vi "Generate API VI.vi"(7 "Highlight changes?":bool=TRUE, 8 "error in (no error)":errorcluster, 9 "class path":path, 10 "API Message":string) -> (0 "error out":errorcluster)   [LabVIEW 2020, in "Method Generation.lvlib" / "API VI Generator.lvclass"]
uses:
  API VI Generator.lvclass
  API VI Generator.lvclass/API VI Generator.ctl
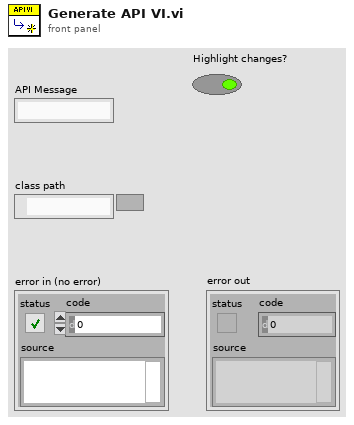
[diagram p1: front panel]
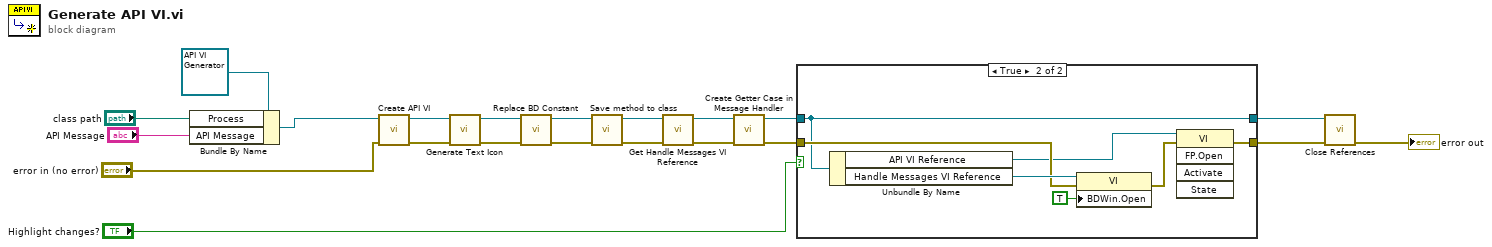
[diagram p0: block diagram]
diagram:
  n1 = Bundle By Name(cluster=refnum<class "API VI Generator.lvclass"> refnum ("New Getter Dialog In"), "Process"="class path", "API Message"="API Message") -> (w17:refnum<class "API VI Generator.lvclass">)
  n2 = call "Create API VI.vi"("error in (no error)"="error in (no error)", "Setter Generator In"=w17) -> ("error out"=w21:errorcluster, "Setter Generator Out"=w2:refnum<class "API VI Generator.lvclass">)  [unwired: 8 in]
  n3 = call "Generate Text Icon.vi"("error in (no error)"=w21, "API VI Generator In"=w2) -> ("error out"=w3:errorcluster, "API VI Generator Out"=w1:refnum<class "API VI Generator.lvclass">)  [unwired: 8 in]
  n4 = call "Replace BD Constant.vi"("error in (no error)"=w3, "Setter Generator In"=w1) -> ("error out"=w14:errorcluster, "Setter Generator Out"=w13:refnum<class "API VI Generator.lvclass">)  [unwired: 8 in]
  n5 = call "Save method to class.vi"("error in (no error)"=w14, "Setter Generator In"=w13) -> ("error out"=w10:errorcluster, "Setter Generator Out"=w11:refnum<class "API VI Generator.lvclass">)  [unwired: 8 in]
  n6 = call "Get Handle Messages VI Reference.vi"("error in (no error)"=w10, "Setter Generator In"=w11) -> ("error out"=w12:errorcluster, "Setter Generator Out"=w9:refnum<class "API VI Generator.lvclass">)  [unwired: 8 in]
  n7 = call "Create Getter Case in Message Handler.vi"("error in (no error)"=w12, "Setter Generator In"=w9) -> ("error out"=w8:errorcluster, "Setter Generator Out"=w5:refnum<class "API VI Generator.lvclass">)  [unwired: 8 in]
  n8 = case shown="True" "Highlight changes?" {
    tunnel: w5 -> [w22 w24]
    tunnel: w8 -> [w23 w28]
    tunnel: [w23 w26] -> w7
    tunnel: [w22 w24] -> w4
    frame False {
    }
    frame True {
      n9 = Unbundle By Name(w24) -> ("API VI Reference"=w25:refnum<vi>, "Handle Messages VI Reference"=w30:refnum<vi>)
      n10 = property class="VI"(reference=w30, error in=w28, "BDWin.Open"=TRUE ("Block Diagram Window:Open")) -> (error out=w27:errorcluster)  [unwired: 1 out]
      n11 = invoke class="VI" method="FP.Open"(reference=w25, error in=w27) -> (error out=w26:errorcluster)  [unwired: 3 in, 4 out]
    }
  }
  n12 = call "Close References.vi"("error in (no error)"=w7, "Setter Generator In"=w4) -> ("error out"=→"error out":errorcluster)  [unwired: 9 in]
